vi "_Read.vi"(8 "error in (no error)":errorcluster, 11 "Level Meter in":refnum<class "Level Meter.lvclass">) -> (0 "error out":errorcluster, 2 "X array":T1, 3 "Level Meter out":refnum<class "Level Meter.lvclass">)   [LabVIEW 2012, in "Level Meter.lvclass"]
doc: "(Protected, Dynamic, Pure Virtual/Abstract) Perform a measurement and return one or more channels of data. Outsiders should not call this method, but instead the public \"Read Data.vi\"."
uses:
  Level Meter.lvclass
  Utility Classes/Readable/X array.ctl
  Utility Classes/Readable/X.ctl
  Level Meter.lvclass/Level Meter.ctl
  Utility Classes/Readable/Readable.lvclass
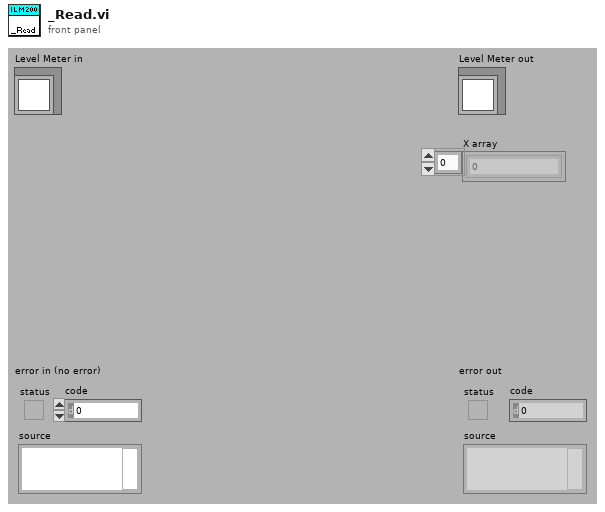
[diagram p1: front panel]
types:
  T1 = typedef "Readable.lvclass/X array.ctl" = T2[]
  T2 = typedef "Readable.lvclass/X.ctl" = dbl
  T3 = typedef "OxfordAddress.ctl" = cluster{"Com Port":i32, "ISOBUS Address":i32, "GPIB Address":i16, "Communication":enum16{"RS232", "ISOBUS", "GPIB", "Gateway"}}
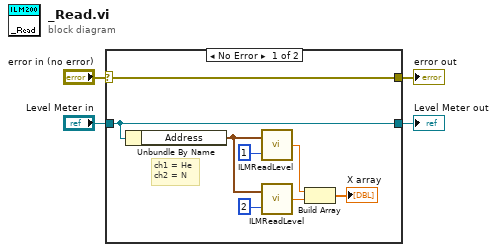
[diagram p0: block diagram]
diagram:
  n1 = case shown="No Error" "error in (no error)" {
    selector: "error in (no error)" -> [w5 w14]
    tunnel: "Level Meter in" -> [w6 w13]
    tunnel: [w6 w13] -> w3
    tunnel: [w5 w14] -> w1
    frame No Error {
      # "ch1 = He\nch2 = N"
      n2 = Unbundle By Name(w6) -> ("Address"=w10:T3)
      n3 = call "ILMReadLevel.vi"("Address"=w10, "Channel number (1-3)"=1) -> ("Level"=w9:dbl)  [unwired: 2 out]
      n4 = call "ILMReadLevel.vi"("Address"=w10, "Channel number (1-3)"=2) -> ("Level"=w7:dbl)  [unwired: 2 out]
      n5 = Build Array(w9, w7) -> (→"X array":dbl[])
    }
    frame Error {
    }
  }
  "error out" <- w1
  "Level Meter out" <- w3
